vi "Ex11.vi"() -> ()   [LabVIEW 2016]
panel:
  out "Elapsed Time (s)":dbl caption="경과 시간(초)"
  out "웨이브폼 차트":dbl(graph)
  in  "Stop Time":dbl
  in  "Start Time":dbl
  # "초"
  # "초"
  # "Ex) start 시간 : 2초, Stop 시간 5초 라면, 2초지난 후 차트가 그려지기 시작하고 5초가 되는 순간 끝납니다."
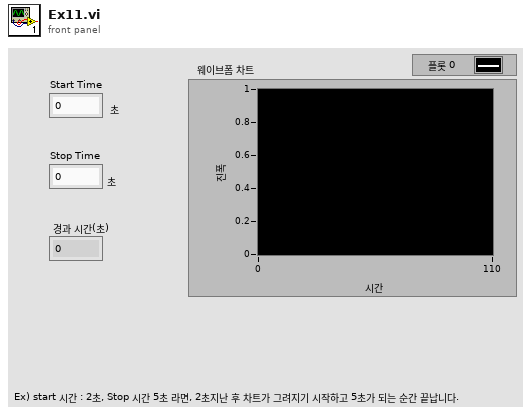
[diagram p1: front panel]
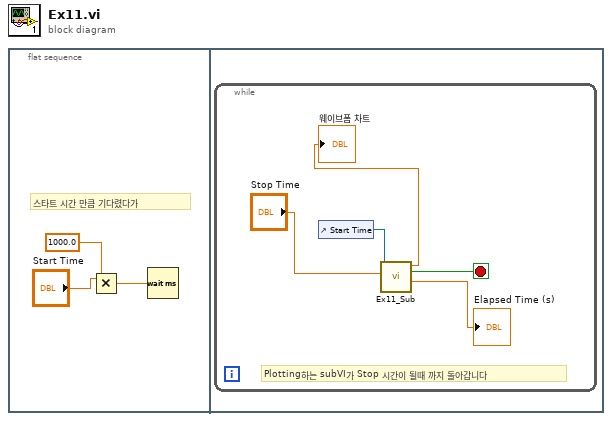
[diagram p0: block diagram]
diagram:
  n1 = flat-sequence {
    frame #0 {
      # "스타트 시간 만큼 기다렸다가"
      n2 = Multiply(x="Start Time", y=1000.0) -> (x*y=w2:dbl)
      n3 = Wait (ms)(milliseconds to wait=w2) -> ()  [unwired: 1 out]
    }
    frame #1 {
      n4 = while {
        stop <- w7 stop-if-true
        # "Plotting하는 subVI가 Stop 시간이 될때 까지 돌아갑니다"
        n5 = control-ref of="Start Time"() -> (w6:refnum<vi>)
        n6 = call "Ex11_Sub.vi"("Stop Time"="Stop Time", "Digital 입력"=w6) -> ("Elapsed Time (s)"=→"Elapsed Time (s)":dbl, "Time has Elapsed"=w7:bool, "웨이브폼 차트"=→"웨이브폼 차트":dbl)  [unwired: 7 in]
      }
    }
  }
